vi "LC_PV_main.vi"() -> ()   [LabVIEW 2016]
uses:
  LC_PV_global.vi
  <vilib>/ErrorRing/Error Ring.xnode
panel:
  out "Weekday_weekend":dbl
  out "OS SubVI Iterations":i16=1304
  in  "RESET OS":bool caption="Reset Outstation"
  in  "ENABLE OS":bool=TRUE
  out "OS SETTINGS CHANGED":bool
  out "MS POLLING? IND":bool=TRUE
  in  "Settings Cluster":T1={"Default Variation:Analog Input Event (OBJ32)"=1, "Default Variation:Analog Input (OBJ30)"=1, "Default Variation:Binary Input (OBJ01)"=1, "Default Variation:Analog Output (OBJ40)"=4, "Default Variation:Binary Output Event (OBJ11)"=1, "Default Variation:Binary Output (OBJ10)"=1, "Default Variation:Analog Output Event (OBJ42)"=8, "Unsolicited Response Allowed"=FALSE, "Control:Select Timeout (ms)"=0, "Misc:Appl Confirmation Timeout"=0} {"Default Variation:Analog Output Event (OBJ42)" items=["32-bit without Time"=1, "16-bit without Time"=2, "32-bit with Time"=3, "16-bit with Time"=4, "Single-prec without Time"=5, "Double-prec without Time"=6, "Single-prec with Time"=7, "Double-prec with Time"=8]; "Default Variation:Binary Output (OBJ10)" items=["Packed Format"=1, "Output Status with Flags"=2]; "Default Variation:Binary Output Event (OBJ11)" items=["Status without Time"=1, "Status with Time"=2]; "Default Variation:Analog Output (OBJ40)" items=["32-bit with Flag"=1, "16-bit with Flag"=2, "Single-prec with Flag"=3, "Double-prec with Flag"=4]; "Default Variation:Binary Input (OBJ01)" items=["Packed Format"=1, "With Flags"=2]; "Default Variation:Analog Input (OBJ30)" items=["32-bit with Flag"=1, "16-bit with Flag"=2, "32-bit without Flag"=3, "16-bit without Flag"=4, "Single-prec with Flag"=5, "Double-prec with Flag"=6]; "Default Variation:Analog Input Event (OBJ32)" items=["32-bit without Time"=1, "16-bit without Time"=2, "32-bit with Time"=3, "16-bit with Time"=4, "Single-prec without Time"=5, "Double-prec without Time"=6, "Single-prec with Time"=7, "Double-prec with Time"=8]}
  in  "Network Settings 1":T2={"port (20000)"=18000, "Master IP"="48.26.87.212", "Master Address"=12340, "Outstation Address "=54320, " update rate"=50}
  in  "DNP3 DataMap 1":T3={"Binary Output Points"=1, "Binary Input Points"=0, "Analog Output Points"=6, "Analog Input Points"=8}
  out "weather":dbl=1.0
  out "PV_manually":bool=TRUE
  out "error out 4":errorcluster
  out "Waveform Chart":dbl(graph)=0.005523681640625
  out "x-y":dbl
  in  "x*y":dbl
  out "MGCC_to_PV":dbl[](array[numeric])=[1.0, 0.0, 0.0, 0.0, 1.0]
  out "appended array":dbl[](array[numeric])=[1.0, 0.0, 0.0, 0.005523681640625, 53.744964599609375, 1.0]
  out "PV_Start_Stop_Cmd":bool=TRUE
  out "error out 3":errorcluster
  out "error out 2":errorcluster
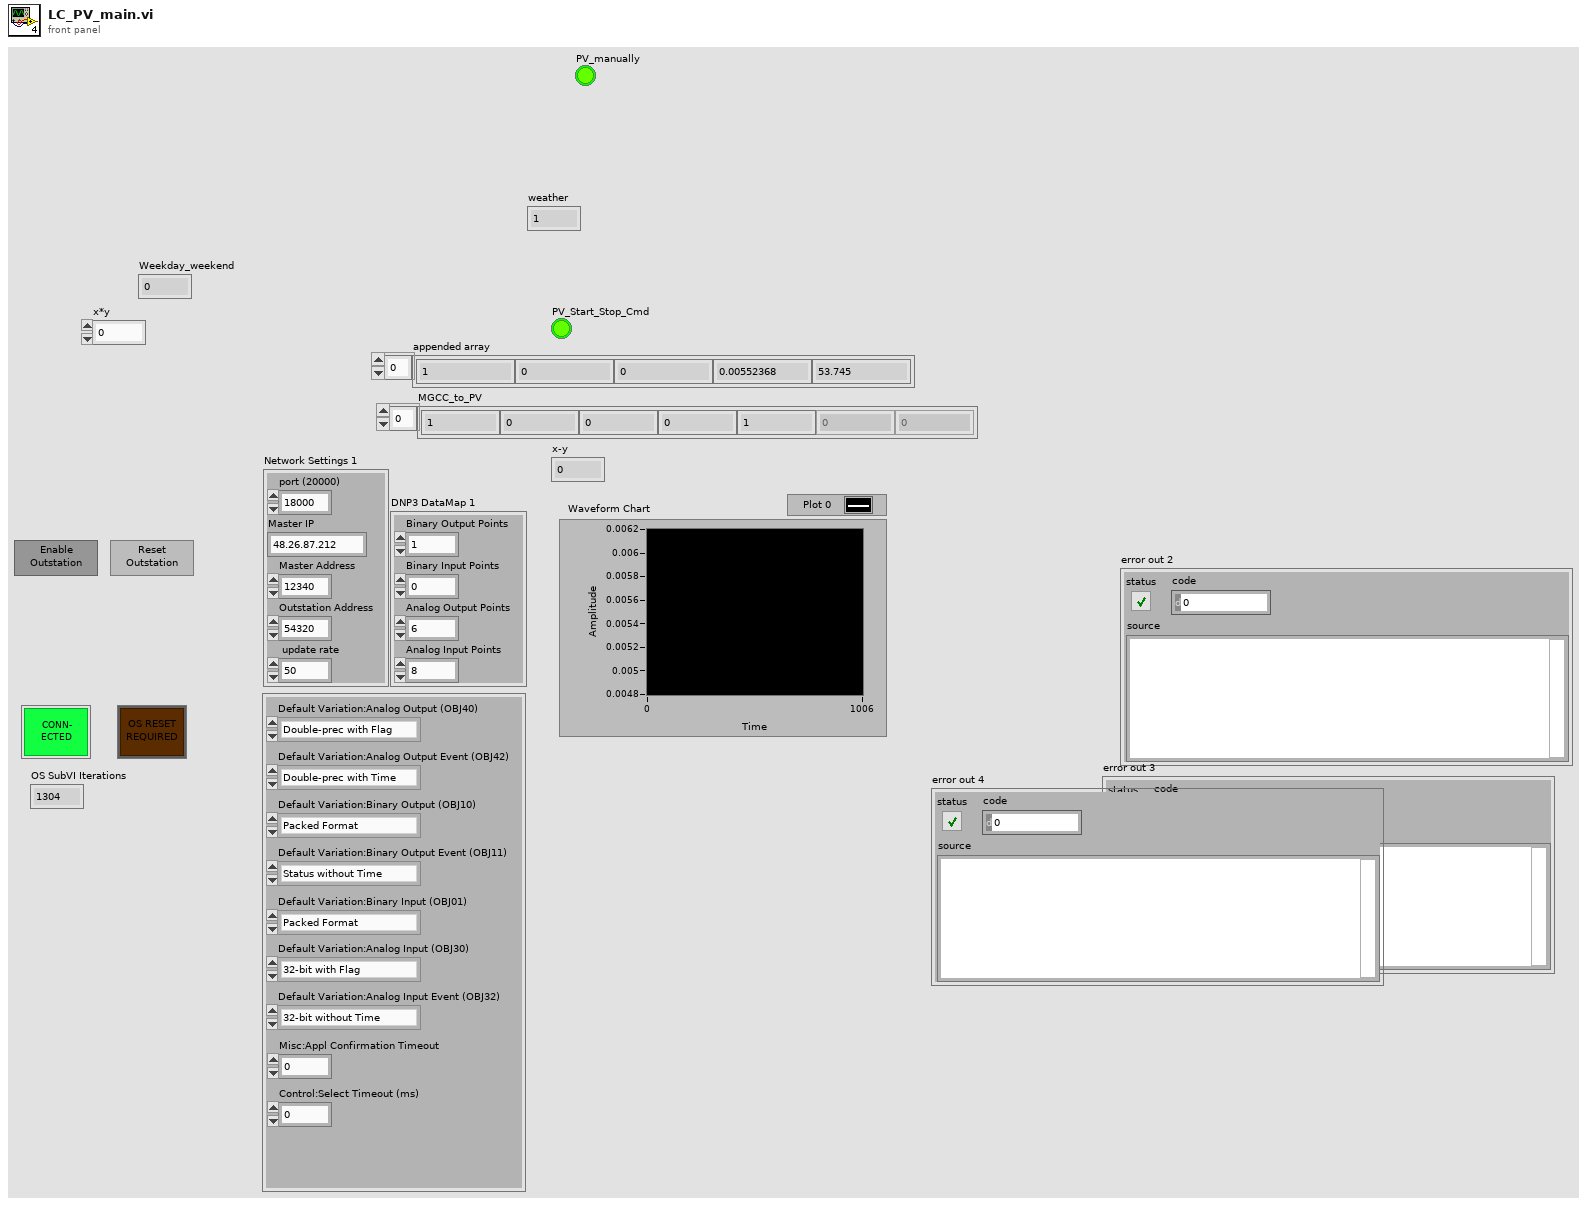
[diagram p1: front panel]
types:
  T1 = cluster{"Default Variation:Analog Input Event (OBJ32)":u8, "Default Variation:Analog Input (OBJ30)":u8, "Default Variation:Binary Input (OBJ01)":u8, "Default Variation:Analog Output (OBJ40)":u8, "Default Variation:Binary Output Event (OBJ11)":u8, "Default Variation:Binary Output (OBJ10)":u8, "Default Variation:Analog Output Event (OBJ42)":u8, "Unsolicited Response Allowed":bool, "Control:Select Timeout (ms)":u32, "Misc:Appl Confirmation Timeout":u32}
  T2 = cluster{"port (20000)":u16, "Master IP":string, "Master Address":u16, "Outstation Address ":u16, " update rate":u32}
  T3 = cluster{"Binary Output Points":u16, "Binary Input Points":u16, "Analog Output Points":u16, "Analog Input Points":u16}
  T4 = cluster{"DNP3 outstation session out":refnum<k21>, "DNP3 outstation out":refnum<k21>, "error out":errorcluster}
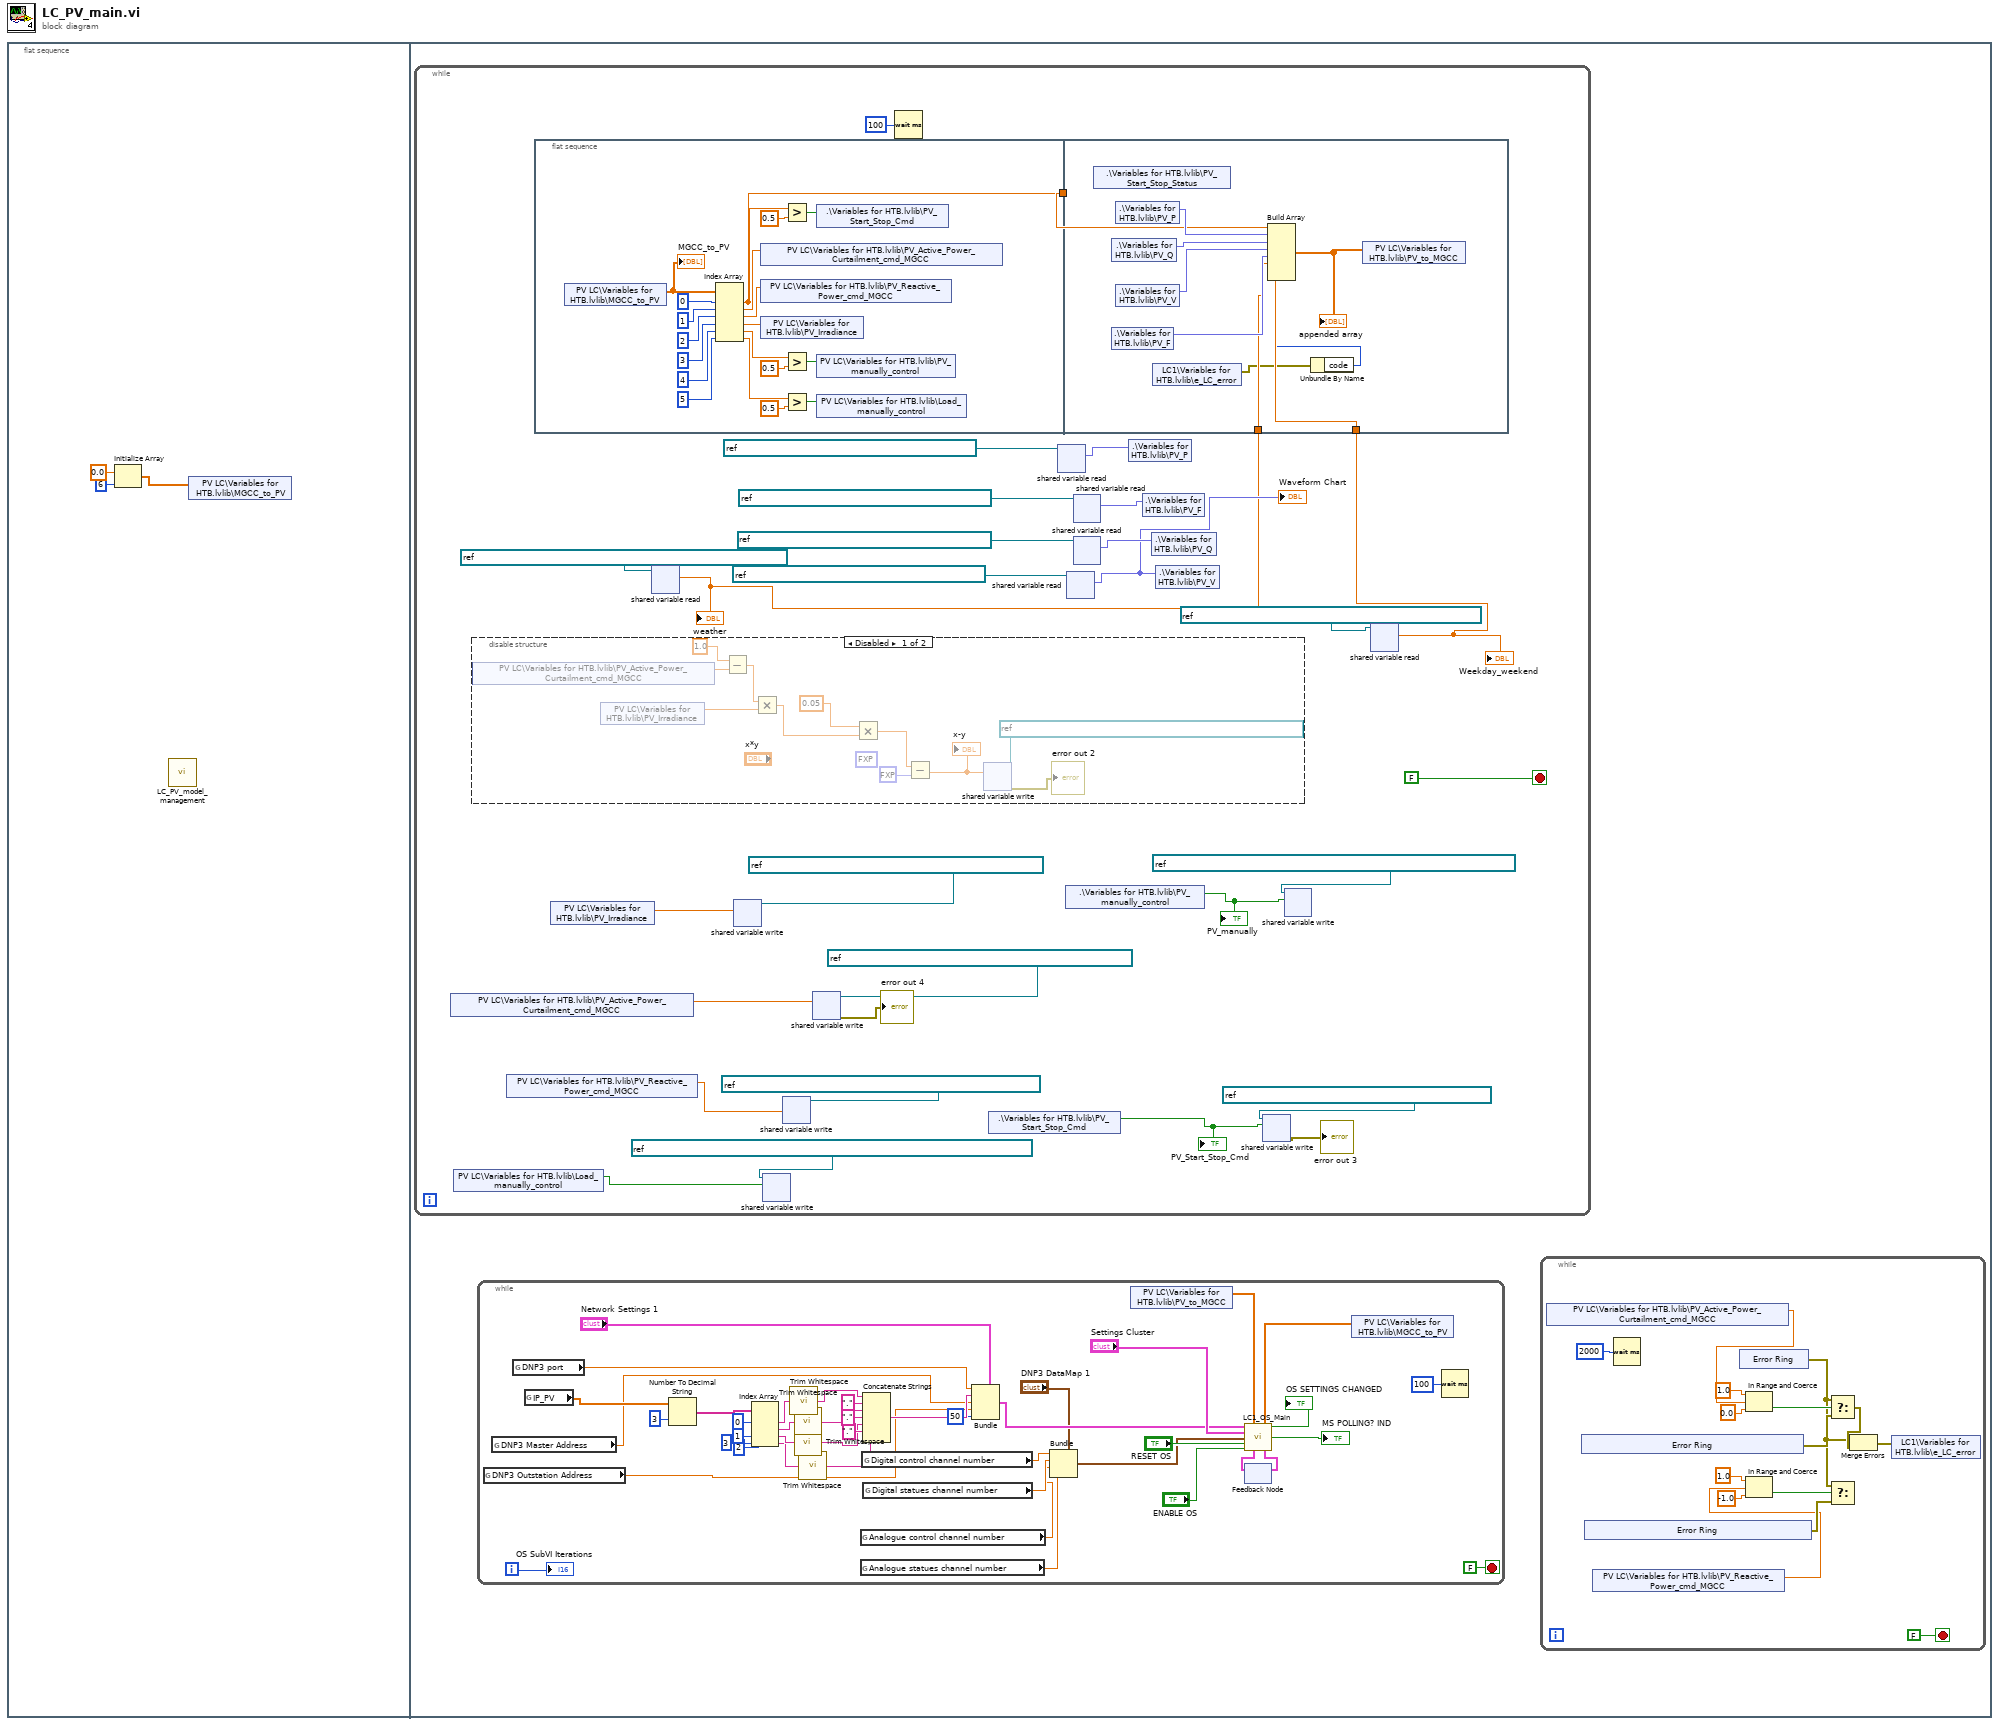
[diagram p0: block diagram]
diagram:
  n1 = flat-sequence {
    frame #0 {
      n2 = Initialize Array(0.0 ("element"), 6 ("dimension size")) -> (w1:dbl[])
      n3 = call "LC_PV_model_management.vi"() -> ()  [unwired: 12 in]
      n4 = shared-variable "PV LC\\Variables for HTB.lvlib\\MGCC_to_PV"(w1) -> ()  [unwired: 1 in, 1 out]
    }
    frame #1 {
      n5 = while {
        stop <- FALSE stop-if-true
        n6 = shared-variable "PV LC\\Variables for HTB.lvlib\\PV_Active_Power_Curtailment_cmd_MGCC"() -> (w75:dbl)  [unwired: 1 in, 1 out]
        n7 = shared-variable "PV LC\\Variables for HTB.lvlib\\Load_manually_control"() -> (w67:bool)  [unwired: 1 in, 1 out]
        n8 = disable-structure shown="Disabled" {
          frame Disabled {
            (unwired) fxp<+/-,64,32> 100.0 ("y")
            n9 = shared-variable "PV LC\\Variables for HTB.lvlib\\PV_Active_Power_Curtailment_cmd_MGCC"() -> (w95:dbl)  [unwired: 1 in, 1 out]
            n10 = shared-variable "PV LC\\Variables for HTB.lvlib\\PV_Irradiance"() -> (w104:dbl)  [unwired: 1 in, 1 out]
            n11 = Subtract(x=1.0, y=w95) -> (x-y=w99:dbl)
            n12 = Multiply(x=w99, y=w104) -> (x*y=w96:dbl)
            n13 = Multiply(x=0.05, y=w96) -> (x*y=w102:dbl)
            n14 = Subtract(x=w102, y=fxp<+/-,64,65> 2.0) -> (x-y=w94:dbl)
            "x-y" <- w94
            n15 = shared-variable-write(refnum<k21> "ni.var.psp://cepd00622/Variables from Host/PV Curtailment" ("shared variable refnum in"), w94) -> (→"error out 2":errorcluster)  [unwired: 1 in, 1 out]
          }
          frame Enabled {
          }
        }
        n16 = shared-variable "PV LC\\Variables for HTB.lvlib\\PV_Reactive_Power_cmd_MGCC"() -> (w78:dbl)  [unwired: 1 in, 1 out]
        n17 = flat-sequence {
          tunnel: [w113] -> w91
          tunnel: w91 -> [w128]
          tunnel: w69 -> [w127]
          tunnel: w65 -> [w126]
          frame #0 {
            n18 = shared-variable "PV LC\\Variables for HTB.lvlib\\MGCC_to_PV"() -> (w123:dbl[])  [unwired: 1 in, 1 out]
            "MGCC_to_PV" <- w123
            n19 = Index Array(array=w123, index #1=0 ("index"), index #2=1 ("index"), index #3=2 ("index"), index #4=3 ("index"), index #5=4 ("index"), index #6=5 ("index")) -> (element #1=w113:dbl, element #2=w116:dbl, element #3=w115:dbl, element #4=w114:dbl, element #5=w110:dbl, element #6=w106:dbl)
            n20 = shared-variable "PV LC\\Variables for HTB.lvlib\\PV_Active_Power_Curtailment_cmd_MGCC"(w116) -> ()  [unwired: 1 in, 1 out]
            n21 = shared-variable "PV LC\\Variables for HTB.lvlib\\PV_Reactive_Power_cmd_MGCC"(w115) -> ()  [unwired: 1 in, 1 out]
            n22 = shared-variable "PV LC\\Variables for HTB.lvlib\\PV_Irradiance"(w114) -> ()  [unwired: 1 in, 1 out]
            n23 = Greater?(x=w113, y=0.5) -> (0:w117:bool)
            n24 = Greater?(x=w110, y=0.5) -> (0:w109:bool)
            n25 = Greater?(x=w106, y=0.5) -> (0:w107:bool)
            n26 = shared-variable ".\\Variables for HTB.lvlib\\PV_Start_Stop_Cmd"(w117) -> ()  [unwired: 1 in, 1 out]
            n27 = shared-variable "PV LC\\Variables for HTB.lvlib\\PV_manually_control"(w109) -> ()  [unwired: 1 in, 1 out]
            n28 = shared-variable "PV LC\\Variables for HTB.lvlib\\Load_manually_control"(w107) -> ()  [unwired: 1 in, 1 out]
          }
          frame #1 {
            n29 = shared-variable ".\\Variables for HTB.lvlib\\PV_Start_Stop_Status"() -> ()  [unwired: 1 in, 2 out]
            n30 = shared-variable ".\\Variables for HTB.lvlib\\PV_Q"() -> (w132:fxp<+/-,64,32>)  [unwired: 1 in, 1 out]
            n31 = shared-variable ".\\Variables for HTB.lvlib\\PV_F"() -> (w130:fxp<+/-,64,32>)  [unwired: 1 in, 1 out]
            n32 = shared-variable ".\\Variables for HTB.lvlib\\PV_P"() -> (w133:fxp<+/-,64,32>)  [unwired: 1 in, 1 out]
            n33 = shared-variable ".\\Variables for HTB.lvlib\\PV_V"() -> (w131:fxp<+/-,64,32>)  [unwired: 1 in, 1 out]
            n34 = shared-variable "LC1\\Variables for HTB.lvlib\\e_LC_error"() -> (w125:errorcluster)  [unwired: 1 in, 1 out]
            n35 = Unbundle By Name(w125) -> ("code"=w124:i32)
            n36 = Build Array(w128, w133, w132, w131, w130, w127, w126, w124) -> (w129:dbl[])
            "appended array" <- w129
            n37 = shared-variable "PV LC\\Variables for HTB.lvlib\\PV_to_MGCC"(w129) -> ()  [unwired: 1 in, 1 out]
          }
        }
        n38 = shared-variable "PV LC\\Variables for HTB.lvlib\\PV_Irradiance"() -> (w73:dbl)  [unwired: 1 in, 1 out]
        n39 = shared-variable-read(refnum<k21> "ni.var.psp://cepd00622/Variables for Microgrid/Weather forecast" ("shared variable refnum in")) -> (w69:dbl)  [unwired: 1 in, 2 out]
        "weather" <- w69
        n40 = shared-variable-write(refnum<k21> "ni.var.psp://cepd00622/Variables from Host/PV Irradiance" ("shared variable refnum in"), w73) -> ()  [unwired: 1 in, 2 out]
        n41 = shared-variable-write(refnum<k21> "ni.var.psp://cepd00622/Variables for Microgrid/Load active power manual select" ("shared variable refnum in"), w67) -> ()  [unwired: 1 in, 2 out]
        n42 = shared-variable-write(refnum<k21> "ni.var.psp://cepd00622/Variables from Host/L2 Reactive Power" ("shared variable refnum in"), w78) -> ()  [unwired: 1 in, 2 out]
        n43 = shared-variable-write(refnum<k21> "ni.var.psp://cepd00622/Variables from Host/PV Curtailment" ("shared variable refnum in"), w75) -> (→"error out 4":errorcluster)  [unwired: 1 in, 1 out]
        n44 = Wait (ms)(milliseconds to wait=u32 100) -> ()  [unwired: 1 out]
        n45 = shared-variable ".\\Variables for HTB.lvlib\\PV_Start_Stop_Cmd"() -> (w83:bool)  [unwired: 1 in, 1 out]
        "PV_Start_Stop_Cmd" <- w83
        n46 = shared-variable-read(refnum<k21> "ni.var.psp://cepd00622/Variables from Host/L2 P" ("shared variable refnum in")) -> (w85:fxp<+/-,64,32>)  [unwired: 1 in, 2 out]
        n47 = shared-variable ".\\Variables for HTB.lvlib\\PV_manually_control"() -> (w72:bool)  [unwired: 1 in, 1 out]
        "PV_manually" <- w72
        n48 = shared-variable-read(refnum<k21> "ni.var.psp://cepd00622/Variables from Host/L2 V" ("shared variable refnum in")) -> (w79:fxp<+/-,64,32>)  [unwired: 1 in, 2 out]
        "Waveform Chart" <- w79
        n49 = shared-variable-read(refnum<k21> "ni.var.psp://cepd00622/Variables from Host/L2 F" ("shared variable refnum in")) -> (w84:fxp<+/-,64,32>)  [unwired: 1 in, 2 out]
        n50 = shared-variable-read(refnum<k21> "ni.var.psp://cepd00622/Variables from Host/L2 Q" ("shared variable refnum in")) -> (w86:fxp<+/-,64,32>)  [unwired: 1 in, 2 out]
        n51 = shared-variable ".\\Variables for HTB.lvlib\\PV_P"(w85) -> ()  [unwired: 1 in, 1 out]
        n52 = shared-variable ".\\Variables for HTB.lvlib\\PV_F"(w84) -> ()  [unwired: 1 in, 1 out]
        n53 = shared-variable ".\\Variables for HTB.lvlib\\PV_Q"(w86) -> ()  [unwired: 1 in, 1 out]
        n54 = shared-variable ".\\Variables for HTB.lvlib\\PV_V"(w79) -> ()  [unwired: 1 in, 1 out]
        n55 = shared-variable-write(refnum<k21> "ni.var.psp://cepd00622/Variables from Host/L2 Start" ("shared variable refnum in"), w83) -> (→"error out 3":errorcluster)  [unwired: 1 in, 1 out]
        n56 = shared-variable-write(refnum<k21> "ni.var.psp://cepd00622/Variables from Host/PV Irradiance manual select" ("shared variable refnum in"), w72) -> ()  [unwired: 1 in, 2 out]
        n57 = shared-variable-read(refnum<k21> "ni.var.psp://cepd00622/Variables for Microgrid/DayofWeek" ("shared variable refnum in")) -> (w65:dbl)  [unwired: 1 in, 2 out]
        "Weekday_weekend" <- w65
      }
      n58 = while {
        i -> [w59]
        stop <- FALSE stop-if-true
        n59 = global read "LC_PV_global.vi" "DNP3 Outstation Address"() -> (w30:dbl)
        n60 = global read "LC_PV_global.vi" "DNP3 Master Address"() -> (w31:dbl)
        n61 = global read "LC_PV_global.vi" "DNP3 port"() -> (w32:dbl)
        n62 = global read "LC_PV_global.vi" "IP_PV"() -> (w34:dbl[])
        n63 = Number To Decimal String(number=w34, width (-)=i16 3) -> (decimal integer string=w51:string[])
        n64 = Index Array(array=w51, index #1=0 ("index"), index #2=1 ("index"), index #3=2 ("index"), index #4=3 ("index")) -> (element #1=w43:string, element #2=w41:string, element #3=w39:string, element #4=w37:string)
        n65 = call <vilib>:"Trim Whitespace.vi"("string"=w43) -> ("trimmed string"=w42:string)  [unwired: 1 in]
        n66 = call <vilib>:"Trim Whitespace.vi"("string"=w41) -> ("trimmed string"=w40:string)  [unwired: 1 in]
        n67 = call <vilib>:"Trim Whitespace.vi"("string"=w39) -> ("trimmed string"=w38:string)  [unwired: 1 in]
        n68 = call <vilib>:"Trim Whitespace.vi"("string"=w37) -> ("trimmed string"=w36:string)  [unwired: 1 in]
        n69 = global read "LC_PV_global.vi" "Analogue control channel number"() -> (w23:dbl)
        n70 = global read "LC_PV_global.vi" "Analogue statues channel number"() -> (w22:dbl)
        n71 = global read "LC_PV_global.vi" "Digital control channel number"() -> (w25:dbl)
        n72 = Concatenate Strings(w42, "." ("string"), w40, "." ("string"), w38, "." ("string"), w36) -> (w33:string)
        n73 = global read "LC_PV_global.vi" "Digital statues channel number"() -> (w24:dbl)
        n74 = Bundle(cluster="Network Settings 1", "port (20000)"=w32, "Master IP"=w33, "Master Address"=w31, "Outstation Address"=w30, "update rate"=u32 50) -> (w28:T2)
        n75 = Bundle(cluster="DNP3 DataMap 1", "Binary Output Points"=w25, "Binary Input Points"=w24, "Analog Output Points"=w23, "Analog Input Points"=w22) -> (w26:T3)
        n76 = shared-variable "PV LC\\Variables for HTB.lvlib\\PV_to_MGCC"() -> (w53:dbl[])  [unwired: 1 in, 1 out]
        n77 = feedback #1() -> (w57:T4)  [unwired: 1 in]
        n78 = call "LC1_OS_Main.vi"("Network Settings 1"=w28, "Analog Input"=w53, "Settings Cluster"="Settings Cluster", "DNP3 DataMap 1"=w26, "OS_Reset"="RESET OS", "OS_Enable"="ENABLE OS", "DNP3 Session Input"=w57) -> ("Analog Output"=w54:dbl[], "OS_DNP3_Settings_Changed"=→"OS SETTINGS CHANGED":bool, "Connected?"=→"MS POLLING? IND":bool, "DNP3 Session"=w58:T4)  [unwired: 2 in, 3 out]
        n79 = feedback-in #1(w58) -> ()
        n80 = shared-variable "PV LC\\Variables for HTB.lvlib\\MGCC_to_PV"(w54) -> ()  [unwired: 1 in, 1 out]
        n81 = Wait (ms)(milliseconds to wait=u32 100) -> ()  [unwired: 1 out]
        "OS SubVI Iterations" <- w59
      }
      n82 = while {
        stop <- FALSE stop-if-true
        n83 = shared-variable "PV LC\\Variables for HTB.lvlib\\PV_Active_Power_Curtailment_cmd_MGCC"() -> (w5:dbl)  [unwired: 1 in, 1 out]
        n84 = xnode "Error Ring"() -> ("error out"=w15:errorcluster)
        n85 = xnode "Error Ring"() -> ("error out"=w11:errorcluster)
        n86 = shared-variable "PV LC\\Variables for HTB.lvlib\\PV_Reactive_Power_cmd_MGCC"() -> (w4:dbl)  [unwired: 1 in, 1 out]
        n87 = Wait (ms)(milliseconds to wait=u32 2000) -> ()  [unwired: 1 out]
        n88 = xnode "Error Ring"() -> ("error out"=w6:errorcluster)
        n89 = In Range and Coerce(upper limit=1.0, x=w5, lower limit=0.0) -> (In Range?=w16:bool)  [unwired: 1 out]
        n90 = In Range and Coerce(upper limit=1.0, x=w4, lower limit=-1.0) -> (In Range?=w14:bool)  [unwired: 1 out]
        n91 = Select(t=w6, s=w16, f=w15) -> (s? t:f=w7:errorcluster)
        n92 = Select(t=w6, s=w14, f=w11) -> ()  [unwired: 1 out]
        n93 = Merge Errors(w6, w7) -> (w8:errorcluster)
        n94 = shared-variable "LC1\\Variables for HTB.lvlib\\e_LC_error"(w8) -> ()  [unwired: 1 in, 1 out]
      }
    }
  }
